vi "Update View Values.vi"(5 "Display State In":T4={"Current Channels Info"=[], "Help Prefix"="", "Max Display Size"=8, "Max Size"=8, "Show Buttons"=TRUE, "Data Valid"=refnum, "Show Range"=FALSE, "Range Items"=[], "Range Index"=[]} caption="State", 7 "Channels In":T1, 11 "Channels Reference":refnum<vi>) -> ()   [LabVIEW 2021, in "myRIO Channel List.xctl"]
uses:
  <vilib>/myRIO/Common/Express VI Framework/xctls/myRIO Channel List/myRIO Channel List.xctl
  <vilib>/myRIO/Common/Express VI Framework/xctls/myRIO Channel List/State.ctl
  <vilib>/myRIO/Common/Profile Manager Framework/typedefs/Channel Info.ctl
  <vilib>/myRIO/Common/Express VI Framework/typedefs/Data Validate Ref.ctl
  <vilib>/myRIO/Common/Express VI Framework/xctls/myRIO Channel List/Data.ctl
  <vilib>/myRIO/Common/Express VI Framework/xctls/myRIO Channel List/typedefs/Channel Data.ctl
  <vilib>/myRIO/Common/Express VI Framework/xctls/myRIO Channel List/typedefs/Remove Channel.ctl
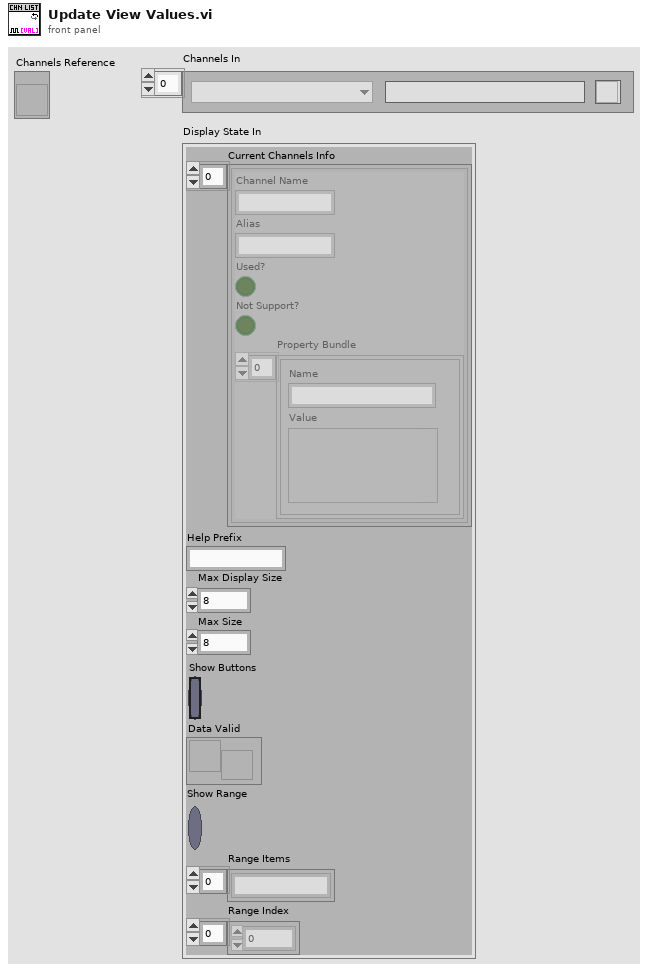
[diagram p1: front panel]
types:
  T1 = typedef "myRIO Channel List.xctl/Data.ctl" = T2[]
  T2 = typedef "myRIO Channel List.xctl/Channel Data.ctl" = cluster{"Channel Name":u16, "Channel Alias":string, "Remove Channel":T3, "Index":i32}
  T3 = typedef "myRIO Channel List.xctl/Remove Channel.ctl" = bool
  T4 = typedef "myRIO Channel List.xctl/State.ctl" = cluster{"Current Channels Info":T5[], "Help Prefix":string, "Max Display Size":i32, "Max Size":i32, "Show Buttons":bool, "Data Valid":T6, "Show Range":bool, "Range Items":string[], "Range Index":i32[]}
  T5 = typedef "Channel Info.ctl" = cluster{"Channel Name":string, "Alias":string, "Used?":bool, "Not Support?":bool, "Property Bundle":cluster{"Name":string, "Value":variant}[]}
  T6 = typedef "Data Validate Ref.ctl" = refnum<user-event>
  T7 = typedef "myRIO Channel List.xctl/Channel View.ctl" = cluster{"Error Icon":T8, "Channel Name":string, "Channel Alias":string, "Remove Channel":T3, "Index":i32, "Range":i32}
  T8 = typedef "myRIO Channel List.xctl/Error Icon.ctl" = bool
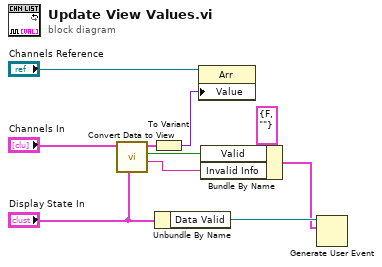
[diagram p0: block diagram]
diagram:
  n1 = call <vilib>:"Convert Data to View.vi"("Display State In"="Display State In", "Channels Data"="Channels In") -> ("Invalid Info"=w1:string, "Data Valid?"=w2:bool, "Channels View Out"=w9:T7[])  [unwired: 7 in]
  n2 = To Variant(anything=w9) -> (Variant=w7:variant)
  n3 = Unbundle By Name("Display State In") -> ("Data Valid"=w5:T6)
  n4 = property class="Arr"(reference="Channels Reference", "Value"=w7) -> ()  [unwired: 1 in, 2 out]
  n5 = Bundle By Name(cluster=cluster{"Valid":bool, "Invalid Info":string} {"Valid"=FALSE, "Invalid Info"=""} ("event data"), "Valid"=w2, "Invalid Info"=w1) -> (w3:cluster{"Valid":bool, "Invalid Info":string})
  n6 = Generate User Event(user event=w5, event data cluster=w3) -> ()  [unwired: 2 in, 2 out]
